vi "DCA Select Instruments to Use.vi"(1 "Instruments on Station":T1[](array[typedef])) -> (0 "Instruments to Use":T2)   [LabVIEW 2011]
uses:
  server/database/Stations/Instruments/Instrument Record.ctl
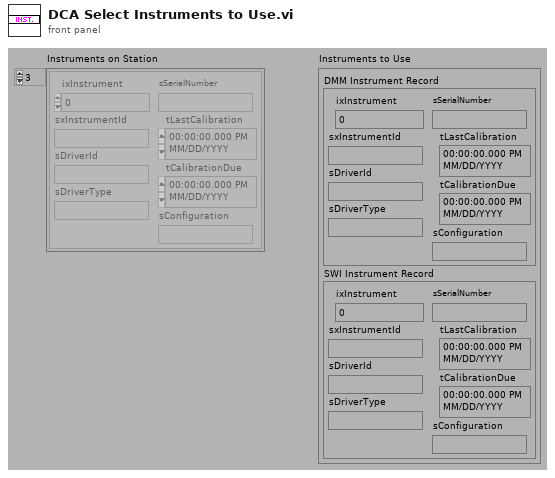
[diagram p1: front panel]
types:
  T1 = typedef "Instrument Record.ctl" = cluster{"ixInstrument":i32, "sxInstrumentId":string, "sDriverId":string, "sDriverType":string, "sSerialNumber":string, "tLastCalibration":timestamp, "tCalibrationDue":timestamp, "sConfiguration":string}
  T2 = cluster{"DMM Instrument Record":T1, "SWI Instrument Record":T1}
  T3 = cluster{"Instrument Information (Cluster)":T1, "Instrument Information (Cluster)":T1}
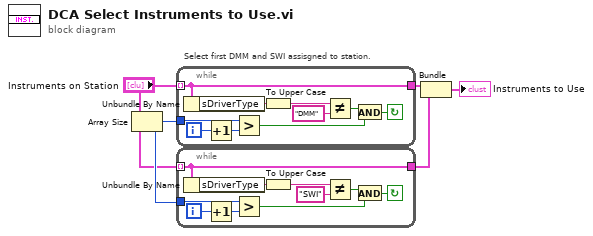
[diagram p0: block diagram]
diagram:
  # "Select first DMM and SWI assisgned to station."
  n1 = Array Size(array="Instruments on Station") -> (size(s)=w4:i32)
  n2 = while {
    tunnel: "Instruments on Station" -> [w12] mode=indexing
    tunnel: [w12] -> w5
    tunnel: w4 -> [w9]
    i -> [w8]
    stop <- w10 continue-if-true
    n3 = Unbundle By Name(w12) -> ("sDriverType"=w15:string)
    n4 = Increment(x=w8) -> (x+1=w6:i32)
    n5 = Greater?(x=w9, y=w6) -> (0:w7:bool)
    n6 = To Upper Case(1:w15) -> (0:w14:string)
    n7 = Not Equal?(x=w14, y="DMM") -> (x != y?=w11:bool)
    n8 = And(x=w11, y=w7) -> (x .and. y?=w10:bool)
  }
  n9 = while {
    tunnel: "Instruments on Station" -> [w22] mode=indexing
    tunnel: [w22] -> w2
    tunnel: w4 -> [w19]
    i -> [w18]
    stop <- w20 continue-if-true
    n10 = Unbundle By Name(w22) -> ("sDriverType"=w25:string)
    n11 = Increment(x=w18) -> (x+1=w16:i32)
    n12 = Greater?(x=w19, y=w16) -> (0:w17:bool)
    n13 = To Upper Case(1:w25) -> (0:w24:string)
    n14 = Not Equal?(x=w24, y="SWI") -> (x != y?=w21:bool)
    n15 = And(x=w21, y=w17) -> (x .and. y?=w20:bool)
  }
  n16 = Bundle("Instrument Information (Cluster)"=w5, "Instrument Information (Cluster)"=w2) -> (→"Instruments to Use":T3)  [unwired: 1 out]
